vi "div.vi"(1 "x2":i16, 2 "x1":i16) -> (0 "y":i16)   [LabVIEW 2018, in "posit.lvlib"]
uses:
  posit.lvlib
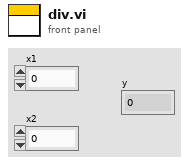
[diagram p1: front panel]
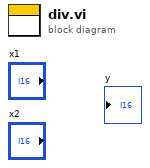
[diagram p0: block diagram]
diagram:
